vi "8P_EnFlo_Specific.vi"(2 "Datalog file path (full)":path, 3 "COM port":refnum<visa-resource-name>, 4 "Log data stream":bool, 5 "Data rate (Hz)":u8(ring)=14 items=["1", "2", "4", "5", "8", "10", "16", "20", "25", "32", "40", "50", "64", "80", "100", "125", "160", "200", "250", "320", "400", "500", "625", "800", "1000"], 6 "N samples":u32=1000, 7 "Command":T2="s") -> (0 "Error":errorcluster, 1 "All samples out":sgl[][](array[numeric]))   [LabVIEW 2017]
uses:
  ctls/Cmd.ctl
panel:
  in  "Main":T1(tab)
  out "Pressure sensor EEPROM checksums ok":bool[](array[boolean])
  out "Pressure sensor temperatures in range":bool[](array[boolean])
  out "Pressure sensor values in range":bool[](array[boolean])
  out "Subsystems ok":bool[](array[boolean])
  out "P_raw_Azero":sgl[](array[numeric])
  out "n":u16
  out "Auto zero progBar":u16(slide) caption="Collecting samples, please maintain dP = 0" scale=0.0..1000.0
  out "Chk ok":bool
  out "EEPROM Checksum":u8 format="%02x"
  in  "EEPROM array":sgl[](array[numeric])
  out "sent":bool
  in  "Stop Data":bool
  out "External thermistor temperature (deg C)":sgl
  out "Checksum ok":bool
  out "Pressures":sgl[][](graph)
  out "Stream enabled":bool
  # "Paul Nathan 08/2017"
  # "Output array order:\nP0......... (Pa)\n.\n.\nP7......... (Pa)\nT_ext.... (deg C)\nT0..........(deg C)\n.\n.\nT7......... (deg C)"
  # "External thermistor value in range"
  # "MCU EEPROM checksum ok"
  # "Pressure sensor 0 EEPROM checksum okay"
  # "Pressure sensor 1 EEPROM checksum okay"
  # "Pressure sensor 2 EEPROM checksum okay"
  # "Pressure sensor 3 EEPROM checksum okay"
  # "Pressure sensor 4 EEPROM checksum okay"
  # "Pressure sensor 5 EEPROM checksum okay"
  # "Pressure sensor 6 EEPROM checksum okay"
  # "Pressure sensor 0 temperature in range"
  # "Pressure sensor 1 temperature in range"
  # "Pressure sensor 2 temperature in range"
  # "Pressure sensor 3 temperature in range"
  # "Pressure sensor 4 temperature in range"
  # "Pressure sensor 5 temperature in range"
  # "Pressure sensor 6 temperature in range"
  # "Pressure sensor 0 value in range"
  # "Pressure sensor 1 value in range"
  # "Pressure sensor 2 value in range"
  # "Pressure sensor 3 value in range"
  # "Pressure sensor 4 value in range"
  # "Pressure sensor 5 value in range"
  # "Pressure sensor 6 value in range"
  # "of 1000"
  # "P0 raw auto-zero"
  # "P1 raw auto-zero"
  # "P2 raw auto-zero"
  # "P3 raw auto-zero"
  # "P4 raw auto-zero"
  # "P5 raw auto-zero"
  # "P6 raw auto-zero"
  # "P7 raw auto-zero"
  # "P0 raw auto-zero"
  # "P1 raw auto-zero"
  # "P2 raw auto-zero"
  # "P3 raw auto-zero"
  # "P4 raw auto-zero"
  # "P5 raw auto-zero"
  # "P6 raw auto-zero"
  # "P7 raw auto-zero"
  # "External thermistor temperature offset (deg C)"
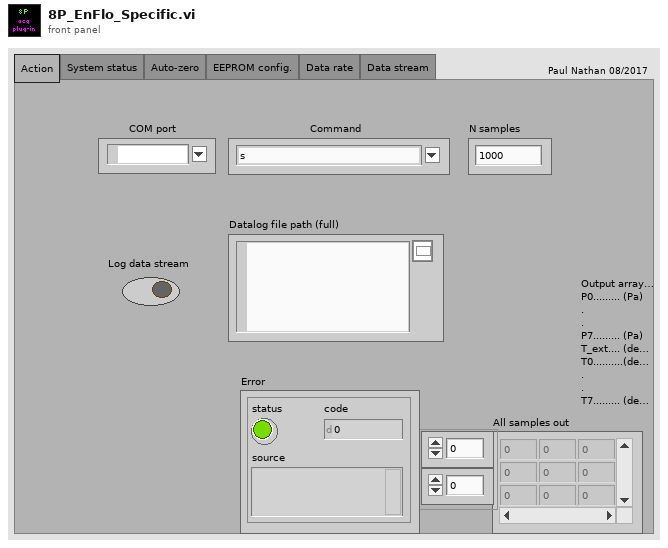
[diagram p1: front panel]
types:
  T1 = enum32{"Action", "System status", "Auto-zero", "EEPROM config.", "Data rate", "Data stream"}
  T2 = typedef "Cmd.ctl" = string
  T3 = enum16{"open", "replace", "create", "open or create", "replace or create", "replace or create with confirmation"}
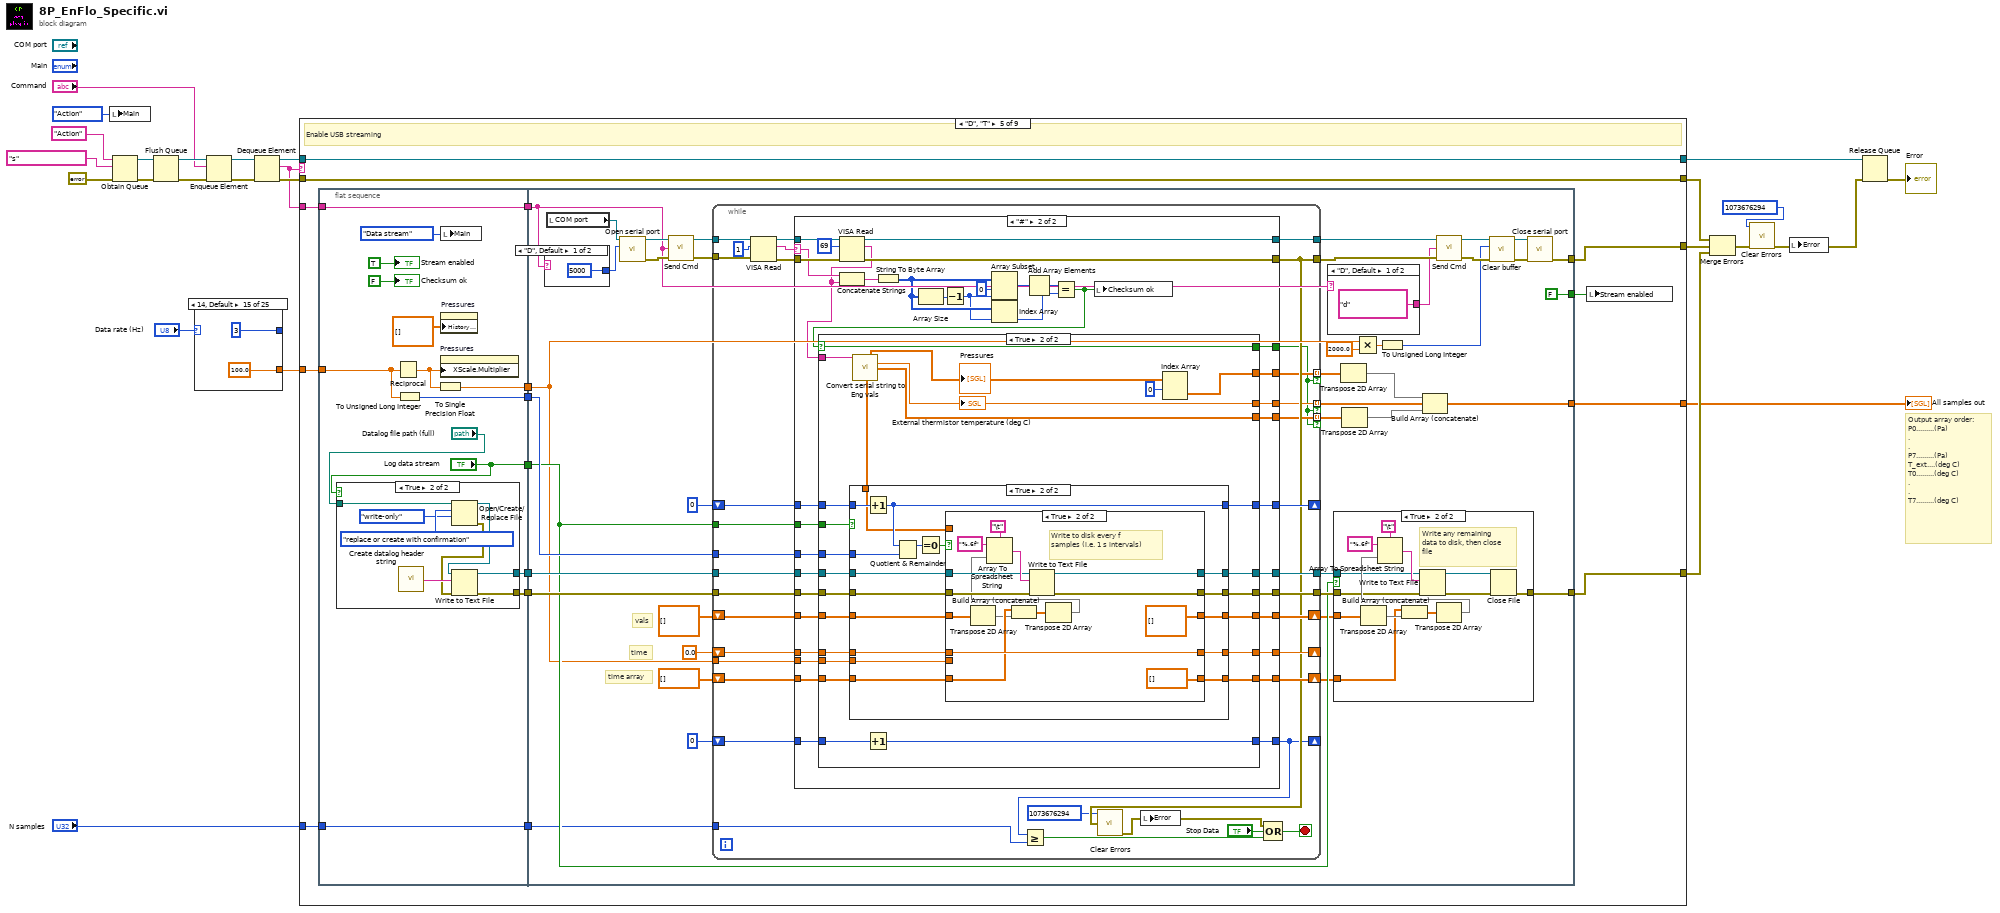
[diagram p0: block diagram]
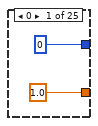
[diagram p2: hidden frame]
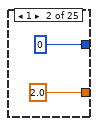
[diagram p3: hidden frame]
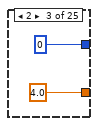
[diagram p4: hidden frame]
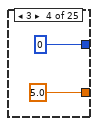
[diagram p5: hidden frame]
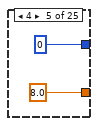
[diagram p6: hidden frame]
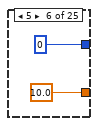
[diagram p7: hidden frame]
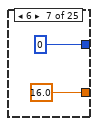
[diagram p8: hidden frame]
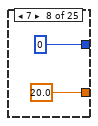
[diagram p9: hidden frame]
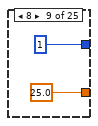
[diagram p10: hidden frame]
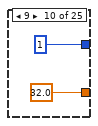
[diagram p11: hidden frame]
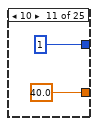
[diagram p12: hidden frame]
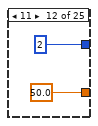
[diagram p13: hidden frame]
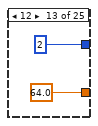
[diagram p14: hidden frame]
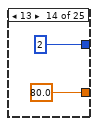
[diagram p15: hidden frame]
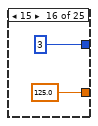
[diagram p16: hidden frame]
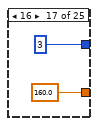
[diagram p17: hidden frame]
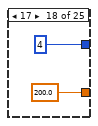
[diagram p18: hidden frame]
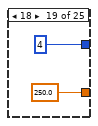
[diagram p19: hidden frame]
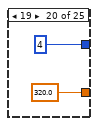
[diagram p20: hidden frame]
diagram:
  # "Output array order:\nP0.........(Pa)\n.\n.\nP7.........(Pa)\nT_ext....(deg C)\nT0.........(deg C)\n.\n.\nT7.........(deg C)"
  n1 = local write "Main"(T1."Action" ("Main")) -> ()
  n2 = Obtain Queue(name (unnamed)="Action", element data type=T2 "s" ("Combo Box"), error in (no error)=errorcluster {"status"=FALSE, "code"=0, "source"=""}) -> (queue out=w24:refnum<queue>, error out=w25:errorcluster)  [unwired: 2 in, 1 out]
  n3 = Flush Queue(queue=w24, error in (no error)=w25) -> (queue out=w22:refnum<queue>, error out=w17:errorcluster)  [unwired: 1 out]
  n4 = case shown="14, Default" "Data rate (Hz)" {
    tunnel: [1.0 2.0 4.0 5.0 8.0 10.0 16.0 20.0 25.0 32.0 40.0 50.0 64.0 80.0 100.0 125.0 160.0 200.0 250.0 320.0 400.0 500.0 625.0 800.0 1000.0] -> w2
    tunnel: [u8 0 u8 0 u8 0 u8 0 u8 0 u8 0 u8 0 u8 0 u8 1 u8 1 u8 1 u8 2 u8 2 u8 2 u8 3 u8 3 u8 3 u8 4 u8 4 u8 4 u8 5 u8 5 u8 6 u8 6 u8 6] -> _
    frame 0 {
    }
    frame 1 {
    }
    frame 2 {
    }
    frame 3 {
    }
    frame 4 {
    }
    frame 5 {
    }
    frame 6 {
    }
    frame 7 {
    }
    frame 8 {
    }
    frame 9 {
    }
    frame 10 {
    }
    frame 11 {
    }
    frame 12 {
    }
    frame 13 {
    }
    frame 14, Default {
    }
    frame 15 {
    }
    frame 16 {
    }
    frame 17 {
    }
    frame 18 {
    }
    frame 19 {
    }
    frame 20 {
    }
    frame 21 {
    }
    frame 22 {
    }
    frame 23 {
    }
    frame 24 {
    }
  }
  n5 = Enqueue Element(queue=w22, element="Command", error in (no error)=w17) -> (queue out=w18:refnum<queue>, error out=w16:errorcluster)  [unwired: 1 in, 1 out]
  n6 = Dequeue Element(queue=w18, error in (no error)=w16) -> (queue out=w13:refnum<queue>, element=w11:T2, error out=w12:errorcluster)  [unwired: 1 in, 1 out]
  n7 = case shown="\"D\", \"T\"" w11 {
    tunnel: w13 -> [w81 w119 w155 w195 w243 w493 w520 w597 w600]
    tunnel: [w81 w119 w155 w195 w243 w493 w520 w597 w600] -> w14
    tunnel: w12 -> [w80 w118 w154 w194 w242 w492 w521 w596 w599]
    tunnel: [w80 w118 w154 w194 w242 w492 w521 w596 w599] -> w10
    tunnel: w11 -> [w79 w117 w153 w193 w241 w495 w518 _ _]
    tunnel: [w77 w115 w151 w190 w239 w494 w516 errorcluster {"status"=FALSE, "code"=0, "source"=""} ("Error out") errorcluster {"status"=FALSE, "code"=0, "source"=""} ("Error out")] -> w9
    tunnel: [_ _ _ _ w238 _ _ _ _] -> w8
    tunnel: w2 -> [_ _ _ _ w234 w491 _ _ _]
    tunnel: "N samples" -> [_ _ _ _ w230 _ _ _ _]
    tunnel: [_ _ _ _ w228 _ _ _ _] -> w4
    frame "S", "s" {
      # "Perform self-test and retrieve status bytes, Retrieve status bytes"
      n8 = flat-sequence {
        tunnel: w79 -> [w84]
        tunnel: [w84] -> w78
        tunnel: w78 -> [w90]
        tunnel: [w85] -> w77
        frame #0 {
          w83 = bool[] [] ("Pressure sensor EEPROM checksums ok")
          n9 = local write "Main"(T1."System status" ("Main")) -> ()
          "Pressure sensor EEPROM checksums ok" <- w83
          "Pressure sensor temperatures in range" <- w83
          "Pressure sensor values in range" <- w83
          "Subsystems ok" <- w83
        }
        frame #1 {
          w94 = 1 ("length (rest)")
          w102 = u8 0 ("byte count")
          n10 = local read "COM port"() -> (w91:refnum<visa-resource-name>)
          n11 = call "Open serial port.vi"("timeout (ms)"=u32 5000, "VISA resource name"=w91) -> ("Error out"=w112:errorcluster, "VISA resource name out"=w113:refnum<visa-resource-name>)  [unwired: 8 in]
          n12 = call "Send Cmd.vi"("Error In"=w112, "Operation"=w90, "Port"=w113) -> ("Error Out"=w110:errorcluster, "Port out"=w111:refnum<visa-resource-name>)  [unwired: 1 in]
          n13 = VISA Read(VISA resource name=w111, byte count=u32 4, error in (no error)=w110) -> (VISA resource name out=w108:refnum<visa-resource-name>, read buffer=w97:string, error out=w107:errorcluster)  [unwired: 1 out]
          n14 = call "Close serial port.vi"("Error in"=w107, "VISA resource name"=w108) -> ("Error out"=w85:errorcluster)  [unwired: 9 in]
          n15 = String Subset(string=w97, offset (0)=0, length (rest)=w94) -> (substring=w106:string)
          n16 = String Subset(string=w97, offset (0)=1, length (rest)=w94) -> (substring=w105:string)
          n17 = String Subset(string=w97, offset (0)=2 ("length (rest)"), length (rest)=w94) -> (substring=w104:string)
          n18 = String Subset(string=w97, offset (0)=3, length (rest)=w94) -> (substring=w103:string)
          n19 = Type Cast(type=w102, x=w106) -> (*(type *) &x=w101:u8)
          n20 = Type Cast(type=w102, x=w105) -> (*(type *) &x=w100:u8)
          n21 = Type Cast(type=w102, x=w104) -> (*(type *) &x=w99:u8)
          n22 = Type Cast(type=w102, x=w103) -> (*(type *) &x=w98:u8)
          n23 = Number To Boolean Array(number=w101) -> (Boolean array=w89:bool[])
          n24 = Number To Boolean Array(number=w100) -> (Boolean array=w88:bool[])
          n25 = Number To Boolean Array(number=w99) -> (Boolean array=w87:bool[])
          n26 = Number To Boolean Array(number=w98) -> (Boolean array=w86:bool[])
          n27 = local write "Pressure sensor EEPROM checksums ok"(w89) -> ()
          n28 = local write "Pressure sensor temperatures in range"(w88) -> ()
          n29 = local write "Pressure sensor values in range"(w87) -> ()
          n30 = local write "Subsystems ok"(w86) -> ()
        }
      }
    }
    frame "Z", "z" {
      # "Perform permanent auto-zero (write values to EEPROM), Perform temporary auto-zero"
      n31 = flat-sequence {
        tunnel: w117 -> [w123]
        tunnel: [w123] -> w116
        tunnel: w116 -> [w130]
        tunnel: [w126] -> w115
        frame #0 {
          n32 = local write "Main"(T1."Auto-zero" ("Main")) -> ()
          "P_raw_Azero" <- sgl[] [] ("P_raw_Azero")
          "Auto zero progBar" <- u16 0 ("Collecting samples, please maintain dP = 0")
        }
        frame #1 {
          n33 = local read "COM port"() -> (w131:refnum<visa-resource-name>)
          n34 = call "Open serial port.vi"("timeout (ms)"=u32 16000, "VISA resource name"=w131) -> ("Error out"=w137:errorcluster, "VISA resource name out"=w138:refnum<visa-resource-name>)  [unwired: 8 in]
          n35 = call "Send Cmd.vi"("Error In"=w137, "Operation"=w130, "Port"=w138) -> ("Error Out"=w135:errorcluster, "Port out"=w136:refnum<visa-resource-name>)  [unwired: 1 in]
          n36 = VISA Read(VISA resource name=w136, byte count=u32 32, error in (no error)=w135) -> (VISA resource name out=w133:refnum<visa-resource-name>, read buffer=w127:string, error out=w132:errorcluster)  [unwired: 1 out]
          n37 = for {
            N: 1000 -> [_]
            shift-right: [w140] -> _
            shift-left: u16 0 -> [w141]
            n38 = Increment(x=w141) -> (x+1=w140:u16)
            "n" <- w140
            n39 = Wait (ms)(milliseconds to wait=u32 11) -> ()  [unwired: 1 out]
            n40 = local write "Auto zero progBar"(w140) -> ()
          }
          n41 = for {
            N: 8 -> [_]
            tunnel: [w144] -> w129 mode=indexing
            tunnel: w127 -> [w143]
            i -> [w150]
            w148 = 4 ("x")
            # "to BE"
            n42 = Multiply(x=w148, y=w150) -> (x*y=w149:i32)
            n43 = String Subset(string=w143, offset (0)=w149, length (rest)=w148) -> (substring=w147:string)
            n44 = Reverse String(1:w147) -> (0:w146:string)
            n45 = Type Cast(type=sgl 0.0 ("byte count"), x=w146) -> (*(type *) &x=w144:sgl)
          }
          n46 = call "Close serial port.vi"("Error in"=w132, "VISA resource name"=w133) -> ("Error out"=w126:errorcluster)  [unwired: 9 in]
          n47 = local write "P_raw_Azero"(w129) -> ()
        }
      }
    }
    frame "R" {
      # "Read all EEPROM values"
      n48 = flat-sequence {
        tunnel: w153 -> [w158]
        tunnel: [w158] -> w152
        tunnel: w152 -> [w172]
        tunnel: [w159] -> w151
        frame #0 {
          n49 = local write "EEPROM array"(sgl[] [] ("EEPROM array")) -> ()
          n50 = local write "Main"(T1."EEPROM config." ("Main")) -> ()
        }
        frame #1 {
          n51 = local read "COM port"() -> (w173:refnum<visa-resource-name>)
          n52 = call "Open serial port.vi"("timeout (ms)"=u32 5000, "VISA resource name"=w173) -> ("Error out"=w179:errorcluster, "VISA resource name out"=w180:refnum<visa-resource-name>)  [unwired: 8 in]
          n53 = call "Send Cmd.vi"("Error In"=w179, "Operation"=w172, "Port"=w180) -> ("Error Out"=w177:errorcluster, "Port out"=w178:refnum<visa-resource-name>)  [unwired: 1 in]
          n54 = VISA Read(VISA resource name=w178, byte count=u32 37, error in (no error)=w177) -> (VISA resource name out=w175:refnum<visa-resource-name>, read buffer=w168:string, error out=w174:errorcluster)  [unwired: 1 out]
          n55 = String To Byte Array(string=w168) -> (unsigned byte array=w162:u8[])
          n56 = call "Close serial port.vi"("Error in"=w174, "VISA resource name"=w175) -> ("Error out"=w159:errorcluster)  [unwired: 9 in]
          n57 = for {
            N: 9 -> [_]
            tunnel: [w185] -> w170 mode=indexing
            tunnel: w168 -> [w184]
            i -> [w189]
            w187 = 4 ("x")
            # "to BE"
            n58 = Multiply(x=w187, y=w189) -> (x*y=w188:i32)
            n59 = String Subset(string=w184, offset (0)=w188, length (rest)=w187) -> (substring=w183:string)
            n60 = Reverse String(1:w183) -> (0:w182:string)
            n61 = Type Cast(type=sgl 0.0 ("byte count"), x=w182) -> (*(type *) &x=w185:sgl)
          }
          n62 = Array Size(array=w162) -> (size(s)=w164:i32)
          n63 = Decrement(x=w164) -> (x-1=w163:i32)
          n64 = Index Array(array=w162, index=36) -> (element=w166:u8)
          n65 = Array Subset(array=w162, index=0, length=w163) -> (w160:u8[])
          n66 = Add Array Elements(numeric array=w160) -> (sum=w161:u8)
          n67 = Equal?(x=w166, y=w161) -> (x = y?=w169:bool)
          n68 = local write "EEPROM array"(w170) -> ()
          n69 = local write "EEPROM Checksum"(w166) -> ()
          n70 = local write "Chk ok"(w169) -> ()
        }
      }
    }
    frame "W" {
      # "Write all EEPROM values (including new checksum)"
      n71 = flat-sequence {
        tunnel: w193 -> [w198]
        tunnel: [w198] -> w192
        tunnel: ["EEPROM array"] -> w191
        tunnel: w192 -> [w213]
        tunnel: w191 -> [w206]
        tunnel: [w199] -> w190
        frame #0 {
          n72 = local write "Main"(T1."EEPROM config." ("Main")) -> ()
        }
        frame #1 {
          n73 = local read "COM port"() -> (w214:refnum<visa-resource-name>)
          n74 = call "Open serial port.vi"("timeout (ms)"=u32 5000, "VISA resource name"=w214) -> ("Error out"=w219:errorcluster, "VISA resource name out"=w220:refnum<visa-resource-name>)  [unwired: 8 in]
          n75 = call "Send Cmd.vi"("Error In"=w219, "Operation"=w213, "Port"=w220) -> ("Error Out"=w217:errorcluster, "Port out"=w218:refnum<visa-resource-name>)  [unwired: 1 in]
          n76 = for {
            N: 9 -> [_]
            tunnel: w206 -> [w224] mode=indexing
            shift-right: [w225] -> w201
            shift-left: "" -> [w226]
            # "to LE"
            n77 = Type Cast(type="", x=w224) -> (*(type *) &x=w223:string)
            n78 = Reverse String(1:w223) -> (0:w222:string)
            n79 = Concatenate Strings(w226, w222) -> (w225:string)
          }
          n80 = String To Byte Array(string=w201) -> (unsigned byte array=w204:u8[])
          n81 = Array Size(array=w204) -> (size(s)=w202:i32)
          n82 = Array Subset(array=w204, index=0, length=w202) -> (w203:u8[])
          n83 = Add Array Elements(numeric array=w203) -> (sum=w200:u8)
          "EEPROM Checksum" <- w200
          n84 = Type Cast(type="", x=w200) -> (*(type *) &x=w209:string)
          n85 = Concatenate Strings(w201, w209) -> (w208:string)
          n86 = VISA Write(VISA resource name=w218, write buffer=w208, error in (no error)=w217) -> (VISA resource name out=w216:refnum<visa-resource-name>, error out=w215:errorcluster)  [unwired: 1 out]
          n87 = call "Close serial port.vi"("Error in"=w215, "VISA resource name"=w216) -> ("Error out"=w199:errorcluster)  [unwired: 9 in]
          "Chk ok" <- TRUE ("Chk ok")
        }
      }
    }
    frame "D", "T" {
      # "Enable USB streaming"
      n88 = flat-sequence {
        tunnel: w241 -> [w257]
        tunnel: [w257] -> w240
        tunnel: [w254] -> w237
        tunnel: [w253] -> w236
        tunnel: [w251] -> w235
        tunnel: w234 -> [w252]
        tunnel: [w249] -> w233
        tunnel: ["Log data stream"] -> w232
        tunnel: w230 -> [w245]
        tunnel: [w245] -> w229
        tunnel: w240 -> [w269]
        tunnel: [w306] -> w239
        tunnel: [w305] -> w238
        tunnel: w237 -> [w302]
        tunnel: w236 -> [w301]
        tunnel: w235 -> [w303]
        tunnel: w233 -> [w282]
        tunnel: w232 -> [w295]
        tunnel: [FALSE] -> w231
        tunnel: w229 -> [w276]
        tunnel: [w273] -> w228
        frame #0 {
          n89 = case shown="True" "Log data stream" {
            tunnel: "Datalog file path (full)" -> [_ w267]
            tunnel: [refnum<file> refnum ("refnum out") w261] -> w254
            tunnel: [errorcluster {"status"=FALSE, "code"=0, "source"=""} ("error out") w260] -> w253
            frame False {
            }
            frame True {
              n90 = call "Create datalog header string.vi"() -> ("Datalog header string"=w263:string)  [unwired: 1 in]
              n91 = Open/Create/Replace File(file path (use dialog)=w267, operation (0:open)=T3."replace or create with confirmation", access (0:read/write)=enum16{"read/write", "read-only", "write-only"}."write-only") -> (refnum out=w264:refnum<file>, error out=w262:errorcluster)  [unwired: 3 in, 1 out]
              n92 = Write to Text File(file (use dialog)=w264, text=w263, error in=w262) -> (refnum out=w261:refnum<file>, error out=w260:errorcluster)  [unwired: 1 in, 1 out]
            }
          }
          n93 = Reciprocal(x=w252) -> (1/x=w250:dbl)
          n94 = To Unsigned Long Integer(number=w252) -> (unsigned 32bit integer=w251:u32)
          n95 = To Single Precision Float(number=w250) -> (single precision float=w249:sgl)
          n96 = property on="Pressures" class="WFChart (strict)"("XScale.Multiplier"=w250) -> ()  [unwired: 2 in, 2 out]
          n97 = local write "Main"(T1."Data stream" ("Main")) -> ()
          n98 = property on="Pressures" class="WFChart (strict)"("History Data"=sgl[][] []) -> ()  [unwired: 2 in, 2 out]
          "Checksum ok" <- FALSE ("Checksum ok")
          "Stream enabled" <- TRUE ("Stream enabled")
        }
        frame #1 {
          # "vals"
          # "time"
          # "time array"
          n99 = case shown="\"D\", Default" w269 {
            tunnel: [u32 5000 ("timeout (ms)") u32 15000 ("timeout (ms)")] -> w308
            frame "D", Default {
            }
            frame "T" {
            }
          }
          n100 = local read "COM port"() -> (w307:refnum<visa-resource-name>)
          n101 = call "Open serial port.vi"("timeout (ms)"=w308, "VISA resource name"=w307) -> ("Error out"=w292:errorcluster, "VISA resource name out"=w294:refnum<visa-resource-name>)  [unwired: 8 in]
          n102 = call "Send Cmd.vi"("Error In"=w292, "Operation"=w269, "Port"=w294) -> ("Error Out"=w291:errorcluster, "Port out"=w293:refnum<visa-resource-name>)  [unwired: 1 in]
          n103 = while {
            tunnel: [w337] -> w289
            tunnel: w293 -> [w339]
            tunnel: [w357] -> w290
            shift-right: [w353] -> _
            shift-left: u32 0 -> [w354]
            tunnel: w303 -> [w352]
            tunnel: w302 -> [w351]
            tunnel: w301 -> [w350]
            tunnel: [w349] -> w300
            tunnel: [w348] -> w299
            shift-right: [w347] -> w279
            shift-left: sgl[][] [] -> [w346]
            shift-right: [w343] -> _
            shift-left: sgl 0.0 ("Numeric") -> [w345]
            tunnel: w282 -> [w344]
            shift-right: [w341] -> w278
            shift-left: sgl[] [] -> [w342]
            tunnel: w295 -> [w340]
            tunnel: w291 -> [w338]
            shift-right: [w331] -> _
            shift-left: u32 0 -> [w334]
            tunnel: w276 -> [w333]
            tunnel: [w330] -> w275 mode=indexing if=w327
            tunnel: [w329] -> w272 mode=indexing if=w327
            tunnel: [w328] -> w271 mode=indexing if=w327
            stop <- w355 stop-if-true
            n104 = VISA Read(VISA resource name=w339, byte count=u32 1, error in (no error)=w338) -> (VISA resource name out=w359:refnum<visa-resource-name>, read buffer=w360:string, error out=w358:errorcluster)  [unwired: 1 out]
            n105 = case shown="\"#\"" w360 {
              selector: w360 -> [_ w403]
              tunnel: w359 -> [w370 w407]
              tunnel: [w371 w405] -> w337
              tunnel: w358 -> [w371 w408]
              tunnel: [w370 w406] -> w357
              tunnel: w354 -> [w369 w393]
              tunnel: [w369 w392] -> w353
              tunnel: w352 -> [_ w391]
              tunnel: w351 -> [w368 w390]
              tunnel: w350 -> [w367 w389]
              tunnel: [w367 w388] -> w349
              tunnel: [w368 w387] -> w348
              tunnel: [w366 w386] -> w347
              tunnel: w346 -> [w366 w385]
              tunnel: w345 -> [w365 w384]
              tunnel: w344 -> [_ w383]
              tunnel: [w365 w382] -> w343
              tunnel: w342 -> [w364 w381]
              tunnel: [w364 w380] -> w341
              tunnel: w340 -> [_ w379]
              tunnel: w334 -> [w363 w377]
              tunnel: [w363 w376] -> w331
              tunnel: [_ w375] -> w330
              tunnel: [FALSE w374] -> w327
              tunnel: [_ w373] -> w329
              tunnel: [_ w372] -> w328
              frame Default {
              }
              frame "#" {
                n106 = VISA Read(VISA resource name=w407, byte count=u32 69, error in (no error)=w408) -> (VISA resource name out=w406:refnum<visa-resource-name>, read buffer=w394:string, error out=w405:errorcluster)  [unwired: 1 out]
                n107 = Concatenate Strings(w403, w394) -> (w395:string)
                n108 = String To Byte Array(string=w395) -> (unsigned byte array=w398:u8[])
                n109 = Array Size(array=w398) -> (size(s)=w401:i32)
                n110 = Decrement(x=w401) -> (x-1=w397:i32)
                n111 = Array Subset(array=w398, index=0, length=w397) -> (w402:u8[])
                n112 = Index Array(array=w398, index=w397) -> (element=w396:u8)
                n113 = Add Array Elements(numeric array=w402) -> (sum=w399:u8)
                n114 = Equal?(x=w399, y=w396) -> (x = y?=w378:bool)
                n115 = case shown="True" w378 {
                  selector: w378 -> [w409 w419]
                  tunnel: w394 -> [_ w441]
                  tunnel: w393 -> [w416 w440]
                  tunnel: [w416 w439] -> w392
                  tunnel: w391 -> [_ w438]
                  tunnel: w390 -> [w415 w436]
                  tunnel: w389 -> [w414 w435]
                  tunnel: [w414 w434] -> w388
                  tunnel: [w415 w433] -> w387
                  tunnel: w385 -> [w413 w432]
                  tunnel: [w413 w431] -> w386
                  tunnel: w384 -> [w412 w430]
                  tunnel: w383 -> [_ w429]
                  tunnel: [w412 w428] -> w382
                  tunnel: w381 -> [w411 w427]
                  tunnel: [w411 w426] -> w380
                  tunnel: w379 -> [_ w425]
                  tunnel: w377 -> [w410 w424]
                  tunnel: [w410 w423] -> w376
                  tunnel: [_ w420] -> w375
                  tunnel: [w409 w419] -> w374
                  tunnel: [_ w418] -> w373
                  tunnel: [_ w417] -> w372
                  frame False {
                  }
                  frame True {
                    n116 = call "Convert serial string to Eng vals.vi"("Serial buffer string (excluding FrameChar)"=w441) -> ("Pressures"=w422:sgl[][], "External thermistor temperature (deg C)"=w418:sgl, "Sensor die temperatures (deg C)"=w417:sgl[], "All vals"=w437:sgl[])  [unwired: 11 in]
                    "Pressures" <- w422
                    "External thermistor temperature (deg C)" <- w418
                    n117 = case shown="True" w425 {
                      tunnel: w440 -> [w447 w464]
                      tunnel: [w447 w463] -> w439
                      tunnel: w438 -> [_ w462]
                      tunnel: w437 -> [_ w459]
                      tunnel: w436 -> [w445 w458]
                      tunnel: w435 -> [w446 w457]
                      tunnel: [w446 w456] -> w434
                      tunnel: [w445 w455] -> w433
                      tunnel: w432 -> [w444 w454]
                      tunnel: [w444 w453] -> w431
                      tunnel: w430 -> [w443 w452]
                      tunnel: w429 -> [_ w451]
                      tunnel: [w443 w450] -> w428
                      tunnel: w427 -> [w442 w449]
                      tunnel: [w442 w448] -> w426
                      frame False {
                      }
                      frame True {
                        n118 = Increment(x=w464) -> (x+1=w463:u32)
                        n119 = Quotient & Remainder(x=w463, y=w462) -> (x-y*floor(x/y)=w461:u32)  [unwired: 1 out]
                        n120 = Equal To 0?(x=w461) -> (x = 0?=w460:bool)
                        n121 = case shown="True" w460 {
                          tunnel: w459 -> [w472 _]
                          tunnel: w458 -> [w473 w486]
                          tunnel: w457 -> [w474 w485]
                          tunnel: [w474 w484] -> w456
                          tunnel: [w473 w483] -> w455
                          tunnel: w454 -> [w466 w478]
                          tunnel: [w465 sgl[][] []] -> w453
                          tunnel: w452 -> [w467 w481]
                          tunnel: w451 -> [w471 _]
                          tunnel: [w470 w481] -> w450
                          tunnel: w449 -> [w469 w480]
                          tunnel: [w468 sgl[] []] -> w448
                          frame False {
                            n122 = Add(x=w467, y=w471) -> (x+y=w470:sgl)
                            n123 = Build Array (concatenate)(w466, w472) -> (w465:sgl[][])
                            n124 = Build Array (concatenate)(w469, w467) -> (w468:sgl[])
                          }
                          frame True {
                            # "Write to disk every f samples (i.e. 1 s intervals)"
                            n125 = Transpose 2D Array(2D array=w478) -> (transposed array=w477:sgl[][])
                            n126 = Build Array (concatenate)(w480, w477) -> (w476:sgl[][])
                            n127 = Transpose 2D Array(2D array=w476) -> (transposed array=w475:sgl[][])
                            n128 = Array To Spreadsheet String(delimiter (Tab)="\t", array=w475, 3:"%.6f" ("format string")) -> (spreadsheet string=w489:string)
                            n129 = Write to Text File(file (use dialog)=w486, text=w489, error in=w485) -> (refnum out=w483:refnum<file>, error out=w484:errorcluster)  [unwired: 1 in, 1 out]
                          }
                        }
                      }
                    }
                    n130 = Increment(x=w424) -> (x+1=w423:u32)
                    n131 = Index Array(array=w422, index (row)=0) -> (element=w420:sgl[])  [unwired: 1 in]
                  }
                }
                n132 = local write "Checksum ok"(w378) -> ()
              }
            }
            n133 = Greater Or Equal?(x=w331, y=w333) -> (x >= y?=w332:bool)
            n134 = call <vilib>:"Clear Errors.vi"("error in (no error)"=w337, "specific error code to clear (0: all)"=1073676294) -> ("error out"=w336:errorcluster)  [unwired: 4 in, 1 out]
            n135 = local write "Error"(w336) -> ()
            n136 = Compound Arithmetic op=OR(w336, "Stop Data", w332) -> (w355:bool)
          }
          n137 = case shown="\"D\", Default" w269 {
            tunnel: [T2 "d" ("Combo Box") T2 "t" ("Combo Box")] -> w268
            frame "D", Default {
            }
            frame "T" {
            }
          }
          n138 = case shown="True" w295 {
            tunnel: [w313 w326] -> w305
            tunnel: w300 -> [w313 w318]
            tunnel: w299 -> [_ w319]
            tunnel: w279 -> [_ w317]
            tunnel: w278 -> [_ w316]
            frame False {
            }
            frame True {
              # "Write any remaining data to disk, then close file"
              n139 = Transpose 2D Array(2D array=w317) -> (transposed array=w323:sgl[][])
              n140 = Build Array (concatenate)(w316, w323) -> (w324:sgl[][])
              n141 = Transpose 2D Array(2D array=w324) -> (transposed array=w325:sgl[][])
              n142 = Array To Spreadsheet String(delimiter (Tab)="\t", array=w325, 3:"%.6f" ("format string")) -> (spreadsheet string=w320:string)
              n143 = Write to Text File(file (use dialog)=w319, text=w320, error in=w318) -> (refnum out=w315:refnum<file>, error out=w314:errorcluster)  [unwired: 1 in, 1 out]
              n144 = Close File(refnum=w315, error in=w314) -> (error out=w326:errorcluster)  [unwired: 1 out]
            }
          }
          n145 = Transpose 2D Array(2D array=w275) -> (transposed array=w274:sgl[][])
          n146 = Transpose 2D Array(2D array=w271) -> (transposed array=w270:sgl[][])
          n147 = Multiply(x=w282, y=sgl 2000.0) -> (x*y=w283:sgl)
          n148 = To Unsigned Long Integer(number=w283) -> (unsigned 32bit integer=w280:u32)
          n149 = Build Array (concatenate)(w274, w272, w270) -> (w273:sgl[][])
          n150 = call "Send Cmd.vi"("Error In"=w289, "Operation"=w268, "Port"=w290) -> ("Error Out"=w286:errorcluster, "Port out"=w287:refnum<visa-resource-name>)  [unwired: 1 in]
          n151 = call "Clear buffer.vi"("Error in"=w286, "dt for timeout (ms)"=w280, "VISA resource name in"=w287) -> ("Error out"=w284:errorcluster, "VISA resource name out"=w285:refnum<visa-resource-name>)  [unwired: 3 in]
          n152 = call "Close serial port.vi"("Error in"=w284, "VISA resource name"=w285) -> ("Error out"=w306:errorcluster)  [unwired: 9 in]
        }
      }
      n153 = local write "Stream enabled"(w231) -> ()
    }
    frame "d", "t" {
      # "Disable USB streaming"
      n154 = flat-sequence {
        tunnel: [w503] -> w496
        tunnel: w495 -> [w503]
        tunnel: w491 -> [w498]
        tunnel: [w497] -> w490
        tunnel: w496 -> [w511]
        tunnel: [w510] -> w494
        tunnel: w490 -> [w505]
        frame #0 {
          n155 = Reciprocal(x=w498) -> (1/x=w500:dbl)
          n156 = disable-structure shown="Disabled" {
            frame Disabled {
              n157 = local write "Main"(T1."Data stream" ("Main")) -> ()
            }
            frame Enabled {
            }
          }
          n158 = To Single Precision Float(number=w500) -> (single precision float=w502:sgl)
          n159 = Multiply(x=w502, y=sgl 2000.0) -> (x*y=w501:sgl)
          n160 = To Unsigned Long Integer(number=w501) -> (unsigned 32bit integer=w497:u32)
        }
        frame #1 {
          n161 = local read "COM port"() -> (w512:refnum<visa-resource-name>)
          n162 = call "Open serial port.vi"("timeout (ms)"=u32 5000, "VISA resource name"=w512) -> ("Error out"=w513:errorcluster, "VISA resource name out"=w514:refnum<visa-resource-name>)  [unwired: 8 in]
          n163 = call "Send Cmd.vi"("Error In"=w513, "Operation"=w511, "Port"=w514) -> ("Error Out"=w509:errorcluster, "Port out"=w507:refnum<visa-resource-name>)  [unwired: 1 in]
          n164 = call "Clear buffer.vi"("Error in"=w509, "dt for timeout (ms)"=w505, "VISA resource name in"=w507) -> ("Error out"=w508:errorcluster, "VISA resource name out"=w506:refnum<visa-resource-name>)  [unwired: 3 in]
          n165 = call "Close serial port.vi"("Error in"=w508, "VISA resource name"=w506) -> ("Error out"=w510:errorcluster)  [unwired: 9 in]
        }
      }
    }
    frame "F" {
      # "Set data rate"
      n166 = flat-sequence {
        tunnel: [w522] -> w519
        tunnel: w518 -> [w522]
        tunnel: w519 -> [w528]
        tunnel: [w526] -> w517
        tunnel: w517 -> [w592]
        tunnel: [w592] -> w516
        frame #0 {
          n167 = local write "Main"(T1."Data rate" ("Main")) -> ()
          n168 = local write "sent"(FALSE ("sent")) -> ()
        }
        frame #1 {
          w530 = ""
          # "to LE"
          n169 = local read "Data rate (Hz)"() -> (w527:u8)
          n170 = case shown="14, Default" w527 {
            tunnel: [1.0 2.0 4.0 5.0 8.0 10.0 16.0 20.0 25.0 32.0 40.0 50.0 64.0 80.0 100.0 125.0 160.0 200.0 250.0 320.0 400.0 500.0 625.0 800.0 1000.0] -> w533
            tunnel: [u8 0 u8 0 u8 0 u8 0 u8 0 u8 0 u8 0 u8 0 u8 1 u8 1 u8 1 u8 2 u8 2 u8 2 u8 3 u8 3 u8 3 u8 4 u8 4 u8 4 u8 5 u8 5 u8 6 u8 6 u8 6] -> w539
            frame 0 {
            }
            frame 1 {
            }
            frame 2 {
            }
            frame 3 {
            }
            frame 4 {
            }
            frame 5 {
            }
            frame 6 {
            }
            frame 7 {
            }
            frame 8 {
            }
            frame 9 {
            }
            frame 10 {
            }
            frame 11 {
            }
            frame 12 {
            }
            frame 13 {
            }
            frame 14, Default {
            }
            frame 15 {
            }
            frame 16 {
            }
            frame 17 {
            }
            frame 18 {
            }
            frame 19 {
            }
            frame 20 {
            }
            frame 21 {
            }
            frame 22 {
            }
            frame 23 {
            }
            frame 24 {
            }
          }
          n171 = local read "COM port"() -> (w525:refnum<visa-resource-name>)
          n172 = To Unsigned Word Integer(number=w533) -> (unsigned 16bit integer=w540:u16)
          n173 = call "Open serial port.vi"("timeout (ms)"=u32 5000, "VISA resource name"=w525) -> ("Error out"=w537:errorcluster, "VISA resource name out"=w538:refnum<visa-resource-name>)  [unwired: 8 in]
          n174 = Type Cast(type=w530, x=w539) -> (*(type *) &x=w541:string)
          n175 = Type Cast(type=w530, x=w540) -> (*(type *) &x=w532:string)
          n176 = Reverse String(1:w532) -> (0:w531:string)
          n177 = Concatenate Strings(w541, w531) -> (w534:string)
          n178 = call "Send Cmd + Data.vi"("Error In"=w537, "Data"=w534, "Operation"=w528, "Port"=w538) -> ("Error Out"=w535:errorcluster, "Port out"=w536:refnum<visa-resource-name>)  [unwired: 1 in]
          n179 = call "Close serial port.vi"("Error in"=w535, "VISA resource name"=w536) -> ("Error out"=w526:errorcluster)  [unwired: 9 in]
        }
        frame #2 {
          n180 = Unbundle By Name(w592) -> ("status"=w594:bool)
          n181 = Not(x=w594) -> (.not. x?=→"sent":bool)
        }
      }
    }
    frame "X" {
      # "Exit"
    }
    frame Default {
    }
  }
  "All samples out" <- w4
  n182 = Merge Errors(w10, w9, w8) -> (w7:errorcluster)
  n183 = call <vilib>:"Clear Errors.vi"("error in (no error)"=w7, "specific error code to clear (0: all)"=1073676294) -> ("error out"=w15:errorcluster)  [unwired: 4 in, 1 out]
  n184 = local write "Error"(w15) -> ()
  n185 = Release Queue(queue=w14, error in (no error)=w15) -> (error out=→"Error":errorcluster)  [unwired: 1 in, 2 out]
